vi "Lectura puerto serial Net Basic.vi"() -> ()   [LabVIEW 2017]
panel:
  out "Read?":bool
  in  "Nombre del puerto":string(combo)
  out "BytesRead":i32
  in  "Read":bool=TRUE
  out "Lectura":string
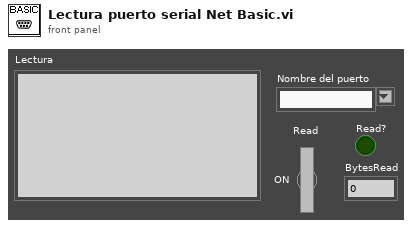
[diagram p1: front panel]
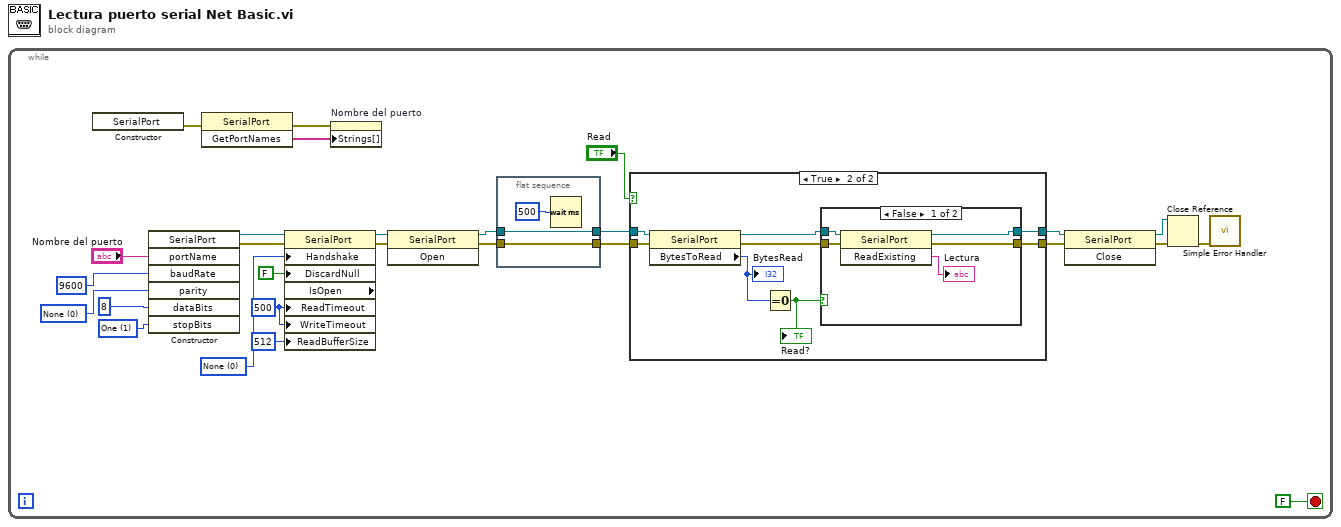
[diagram p0: block diagram]
diagram:
  n1 = while {
    stop <- FALSE stop-if-true
    w5 = 500 ("ReadTimeout")
    w13 = 0 items=["None", "XOnXOff", "RequestToSend", "RequestToSendXOnXOff"] ("Handshake")
    w14 = 1 items=["None", "One", "Two", "OnePointFive"] ("stopBits")
    w16 = 0 items=["None", "Odd", "Even", "Mark", "Space"] ("parity")
    n2 = constructor class="SerialPort"() -> (error out=w3:errorcluster)  [unwired: 3 in, 2 out]
    n3 = constructor class="SerialPort"("portName"="Nombre del puerto", "baudRate"=9600, "parity"=w16, "dataBits"=8, "stopBits"=w14) -> (reference out=w21:refnum<k24>, error out=w18:errorcluster)  [unwired: 3 in, 6 out]
    n4 = invoke class="SerialPort" method="GetPortNames"(error in=w3) -> (error out=w1:errorcluster, "GetPortNames"=w2:string[])  [unwired: 2 in, 1 out]
    n5 = property class="SerialPort" props=["Handshake", "DiscardNull", "IsOpen", "ReadTimeout", "WriteTimeout", "ReadBufferSize"](reference=w21, error in=w18, "Handshake"=w13, "DiscardNull"=FALSE, "ReadTimeout"=w5, "WriteTimeout"=w5, "ReadBufferSize"=512) -> (reference out=w20:refnum<k24>, error out=w19:errorcluster)  [unwired: 1 out]
    n6 = property on="Nombre del puerto" class="CmbBox"(error in=w1, "Strings[]"=w2) -> ()  [unwired: 1 in, 2 out]
    n7 = invoke class="SerialPort" method="Open"(reference=w20, error in=w19) -> (reference out=w11:refnum<k24>, error out=w8:errorcluster)  [unwired: 1 in, 1 out]
    n8 = flat-sequence {
      tunnel: w11 -> [w30]
      tunnel: [w30] -> w10
      tunnel: w8 -> [w29]
      tunnel: [w29] -> w9
      frame #0 {
        n9 = Wait (ms)(milliseconds to wait=u32 500) -> ()  [unwired: 1 out]
      }
    }
    n10 = case shown="True" "Read" {
      tunnel: w10 -> [w32 w40]
      tunnel: w9 -> [w31 w39]
      tunnel: [w32 w36] -> w25
      tunnel: [w31 w35] -> w24
      frame False {
      }
      frame True {
        n11 = property class="SerialPort"(reference=w40, error in=w39) -> (reference out=w38:refnum<k24>, error out=w37:errorcluster, "BytesToRead"=w34:i32)
        "BytesRead" <- w34
        n12 = Equal To 0?(x=w34) -> (x = 0?=w33:bool)
        "Read?" <- w33
        n13 = case shown="False" w33 {
          tunnel: w38 -> [w45 w47]
          tunnel: w37 -> [w44 w46]
          tunnel: [w43 w47] -> w36
          tunnel: [w42 w46] -> w35
          frame False {
            n14 = invoke class="SerialPort" method="ReadExisting"(reference=w45, error in=w44) -> (reference out=w43:refnum<k24>, error out=w42:errorcluster, "ReadExisting"=→"Lectura":string)  [unwired: 1 in]
          }
          frame True {
          }
        }
      }
    }
    n15 = invoke class="SerialPort" method="Close"(reference=w25, error in=w24) -> (reference out=w22:refnum<k24>, error out=w23:errorcluster)  [unwired: 1 in, 1 out]
    n16 = Close Reference(reference=w22, error in (no error)=w23) -> (error out=w27:errorcluster)
    n17 = call <vilib>:"Simple Error Handler.vi"("error in (no error)"=w27) -> ()  [unwired: 1 in, 8 out]
  }
